vi "CalculateResidual.vi"(6 "calc cache":variant, 7 "Feature":T1, 8 "error in (no error)":errorcluster, 9 "Speed (RPM)":dbl, 10 "Channel":T3, 11 "Data":waveform(sgl)) -> (0 "error out":errorcluster, 3 "Residual [EU RMS]":dbl, 4 "calc cache out":variant)   [LabVIEW 2017, in "AnalysisHelper.lvlib"]
uses:
  <vilib>/addons/InsightCM/Utilities/Analysis/Shared/AnalysisHelper.lvlib
  <vilib>/addons/InsightCM/Utilities/Analysis/Shared/controls/Channel.ctl
  <vilib>/addons/InsightCM/Utilities/Analysis/Shared/controls/SpeedType.ctl
  <vilib>/addons/InsightCM/Utilities/Analysis/Shared/controls/Feature.ctl
  <vilib>/addons/InsightCM/Utilities/Analysis/Shared/controls/AmplitudeScale.ctl
  <vilib>/addons/InsightCM/Utilities/Analysis/Shared/controls/BandConfig.ctl
  <vilib>/addons/InsightCM/Utilities/Analysis/Shared/controls/BandDomain.ctl
  <vilib>/addons/InsightCM/Utilities/Analysis/Shared/controls/BandCalculation.ctl
  <vilib>/addons/InsightCM/Utilities/Analysis/Vibration/VibrationAnalysisFunctions.lvlib
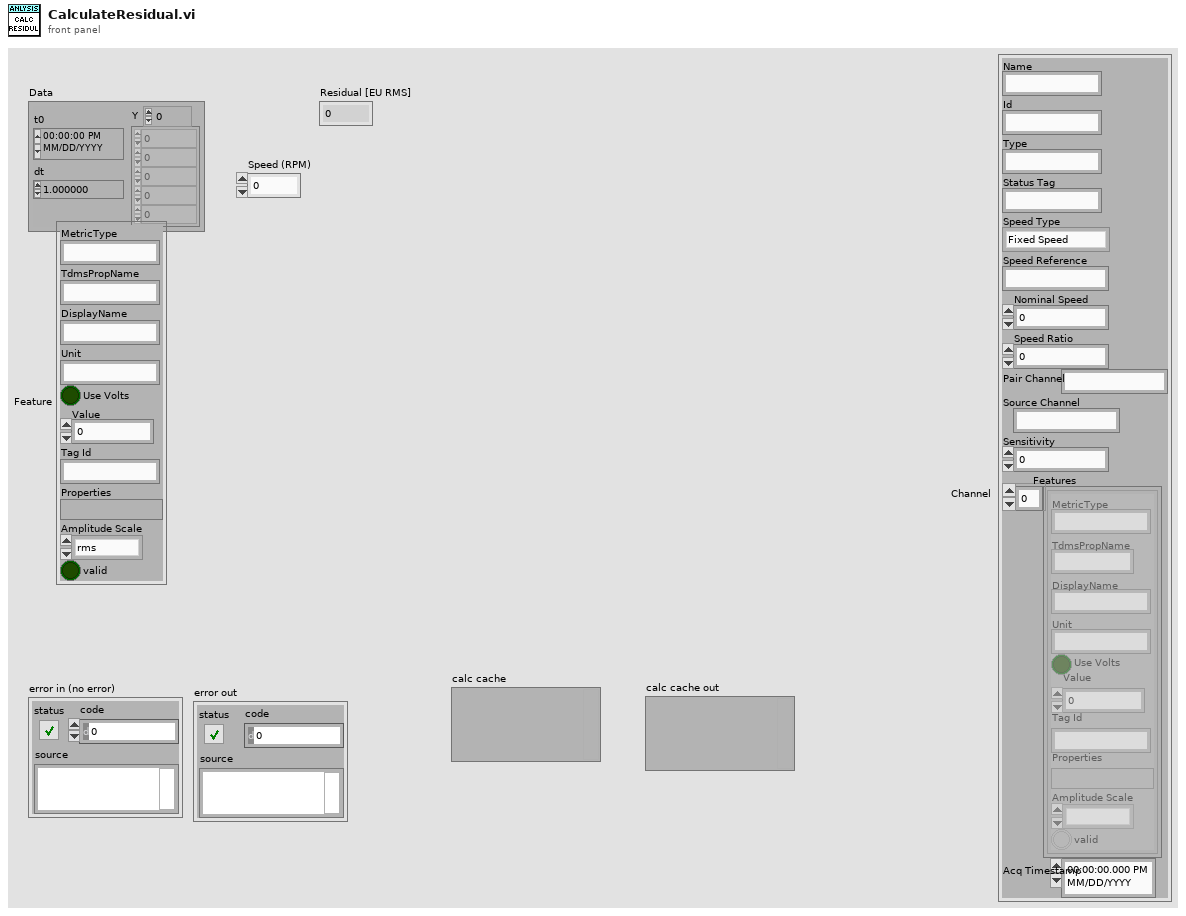
[diagram p1: front panel]
types:
  T1 = typedef "AnalysisHelper.lvlib/Feature.ctl" = cluster{"MetricType":string, "TdmsPropName":string, "DisplayName":string, "Unit":string, "Use Volts":bool, "Value":dbl, "Tag Id":string, "Properties":variant, "Amplitude Scale":T2, "valid":bool}
  T2 = typedef "AnalysisHelper.lvlib/AmplitudeScale.ctl" = enum16{"rms", "peak", "pk-pk"}
  T3 = typedef "AnalysisHelper.lvlib/Channel.ctl" = cluster{"Name":string, "Id":string, "Type":string, "Status Tag":string, "Speed Type":T4, "Speed Reference":string, "Nominal Speed":dbl, "Speed Ratio":dbl, "Pair Channel":string, "Source Channel":string, "Sensitivity":dbl, "Features":T1[], "Acq Timestamp":timestamp}
  T4 = typedef "AnalysisHelper.lvlib/SpeedType.ctl" = enum16{"Fixed Speed", "Tachometer"}
  T5 = typedef "AnalysisHelper.lvlib/BandConfig.ctl" = cluster{"High":dbl, "Low":dbl, "Domain":T6, "Calculation":T7}
  T6 = typedef "AnalysisHelper.lvlib/BandDomain.ctl" = enum16{"Frequency", "CPM", "Orders"}
  T7 = typedef "AnalysisHelper.lvlib/BandCalculation.ctl" = enum16{"Total", "Max", "Phase"}
  T8 = typedef "svc_Spectrum Info.ctl" = cluster{"channel name":string, "description":string, "x-axis units":T9, "spectral info":cluster{"spectrum type":T10, "linear/dB":enum16{"linear", "dB"}, "window":u16, "window size":i32, "FFT size":i32}, "engineering units":T11, "custom label":string, "dB reference [EU]":dbl, "peak units":enum16{"rms", "peak", "peak-peak"}, "weighting filter":T12, "spectral density?":bool, "unit label":string, "spectrum skewed?":bool, "complimentary spectrum units":T13}
  T9 = typedef "svc_X-Axis Units.ctl" = u16
  T10 = typedef "svc_Spectrum Type.ctl" = enum16{"FFT Spectrum [complex]", "Amplitude [Magnitude]", "Power [Magnitude^2]", "Cross Spectrum [complex]", "Frequency Response [Complex]"}
  T11 = typedef "svc_Engineering Units Text Ring.ctl" = u16
  T12 = typedef "svc_Weighting Filter Text Ring.ctl" = u16
  T13 = typedef "svc_Complimentary Spectrum Units.ctl" = enum16{"none", "radians", "degrees", "cycles", "imaginary"}
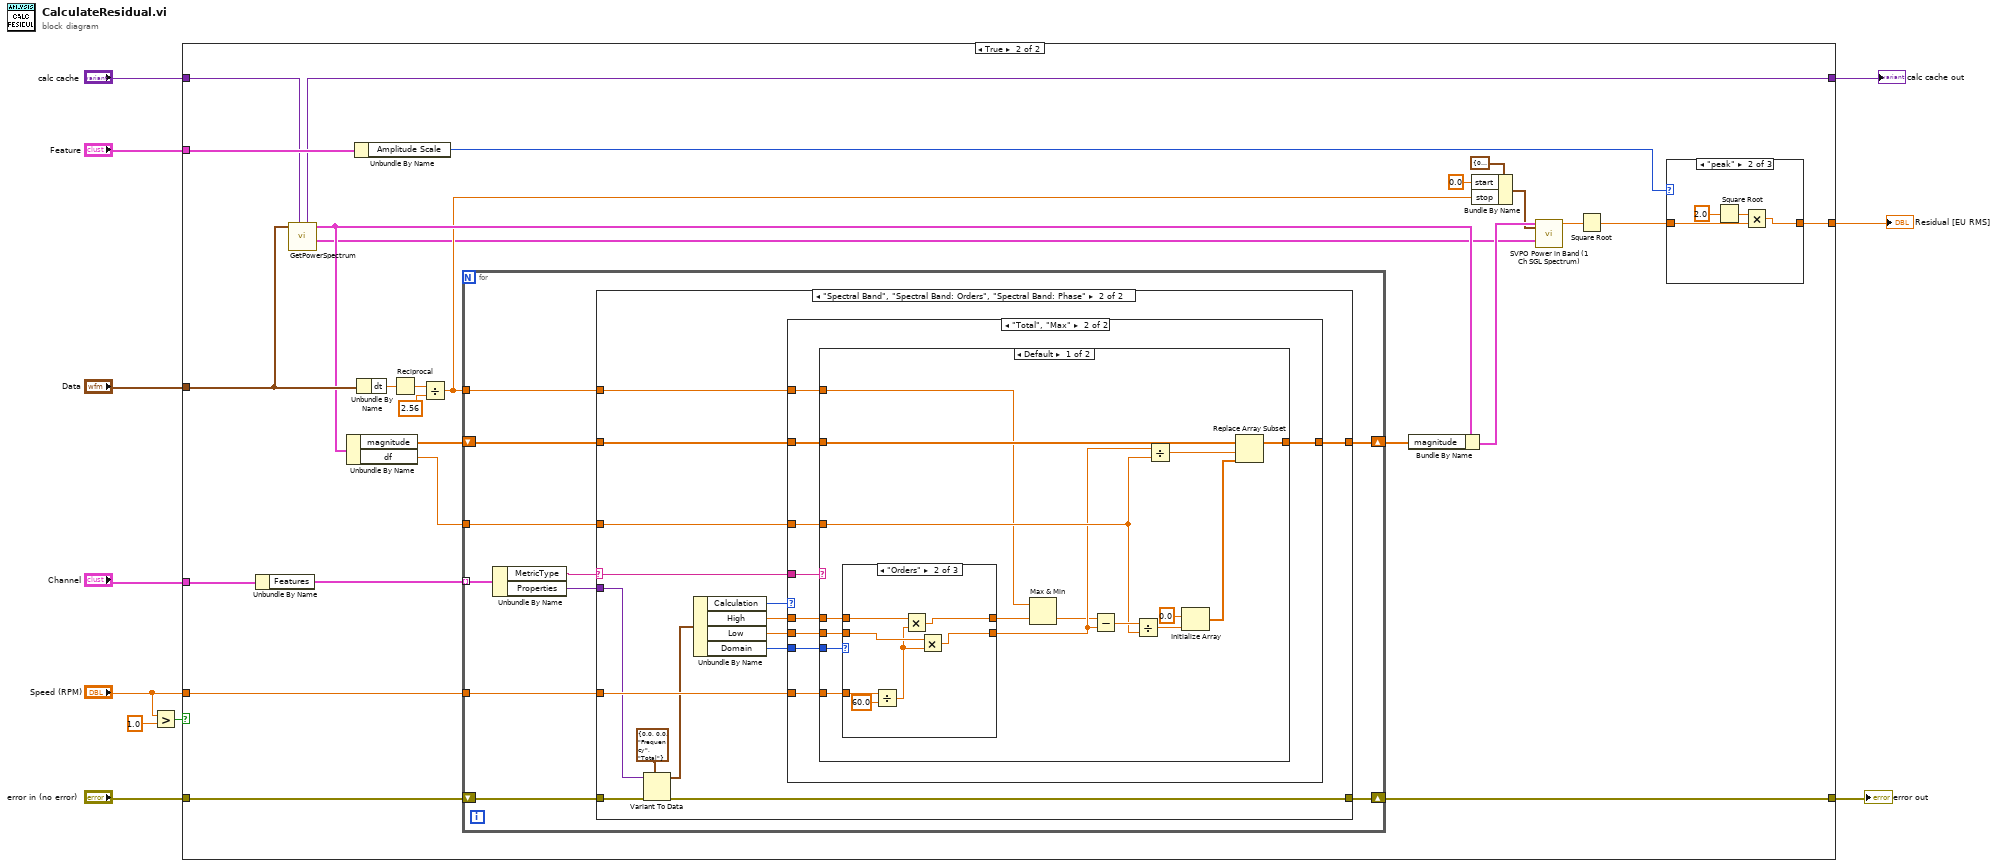
[diagram p0: block diagram]
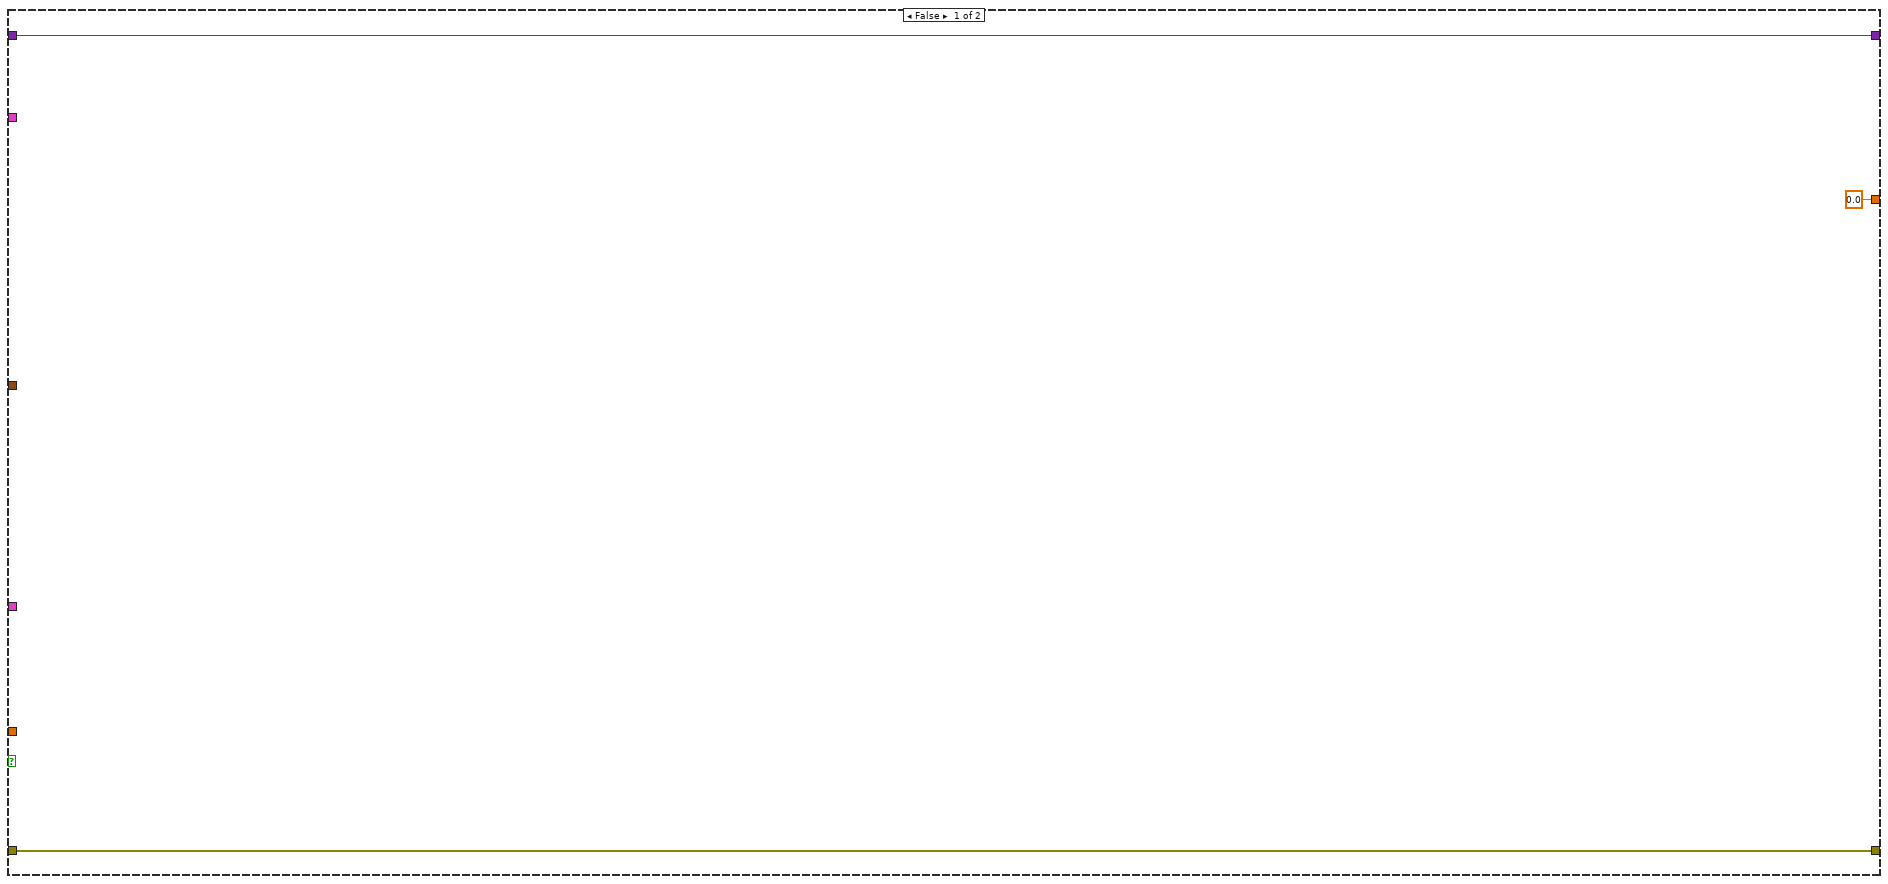
[diagram p2: hidden frame]
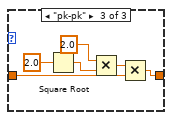
[diagram p4: hidden frame]
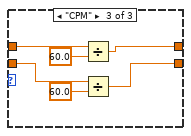
[diagram p8: hidden frame]
diagram:
  n1 = Greater?(x="Speed (RPM)", y=1.0) -> (0:w3:bool)
  n2 = case shown="True" w3 {
    tunnel: "Speed (RPM)" -> [_ w39]
    tunnel: "Data" -> [_ w38]
    tunnel: "error in (no error)" -> [w13 w28]
    tunnel: "Channel" -> [_ w27]
    tunnel: "Feature" -> [_ w25]
    tunnel: [sgl 0.0 w24] -> w7
    tunnel: "calc cache" -> [w12 w18]
    tunnel: [w13 w17] -> w5
    tunnel: [w12 w15] -> w1
    frame False {
    }
    frame True {
      n3 = Unbundle By Name(w27) -> ("Features"=w26:T1[])
      n4 = call <vilib>:"GetPowerSpectrum.vi"("calc cache"=w18, "Waveform"=w38) -> ("spectrum info"=w20:T8, "power spectrum [EU^2 rms]"=w34:cluster{"f0":dbl, "df":dbl, "magnitude":sgl[]}, "calc cache out"=w15:variant)  [unwired: 7 in]
      n5 = Unbundle By Name(w34) -> ("magnitude"=w32:sgl[], "df"=w40:dbl)
      n6 = Unbundle By Name(w25) -> ("Amplitude Scale"=w23:T2)
      n7 = Unbundle By Name(w38) -> ("dt"=w37:dbl)
      n8 = Reciprocal(x=w37) -> (1/x=w36:dbl)
      n9 = Divide(x=w36, y=2.56) -> (x/y=w29:dbl)
      n10 = for {
        tunnel: w26 -> [w61] mode=indexing
        shift-right: [w59] -> w33
        shift-left: w32 -> [w58]
        tunnel: w40 -> [w57]
        tunnel: w39 -> [w56]
        tunnel: w29 -> [w55]
        shift-right: [w53] -> w17
        shift-left: w28 -> [w54]
        n11 = Unbundle By Name(w61) -> ("MetricType"=w60:string, "Properties"=w52:variant)
        n12 = case shown="\"Spectral Band\", \"Spectral Band: Orders\", \"Spectral Band: Phase\"" w60 {
          selector: w60 -> [_ w70]
          tunnel: [w63 w78] -> w59
          tunnel: w58 -> [w63 w77]
          tunnel: w57 -> [_ w76]
          tunnel: w56 -> [_ w75]
          tunnel: w55 -> [_ w74]
          tunnel: w54 -> [w62 w66]
          tunnel: [w62 w65] -> w53
          tunnel: w52 -> [_ w64]
          frame "False", Default {
          }
          frame "Spectral Band", "Spectral Band: Orders", "Spectral Band: Phase" {
            n13 = Variant To Data(error in=w66, type=T5 {"High"=0.0, "Low"=0.0, "Domain"=enum."Frequency", "Calculation"=enum."Total"} ("SpectralBand"), Variant=w64) -> (data=w72:T5, error out=w65:errorcluster)
            n14 = Unbundle By Name(w72) -> ("Calculation"=w71:T7, "High"=w69:dbl, "Low"=w68:dbl, "Domain"=w67:T6)
            n15 = case shown="\"Total\", \"Max\"" w71 {
              tunnel: [w79 w88] -> w78
              tunnel: w77 -> [w79 w87]
              tunnel: w69 -> [_ w86]
              tunnel: w68 -> [_ w85]
              tunnel: w67 -> [_ w84]
              tunnel: w76 -> [_ w83]
              tunnel: w75 -> [_ w82]
              tunnel: w74 -> [_ w81]
              tunnel: w70 -> [_ w80]
              frame "Phase" {
              }
              frame "Total", "Max" {
                n16 = case shown="Default" w80 {
                  tunnel: [w89 w120] -> w88
                  tunnel: w87 -> [w104 w120]
                  tunnel: w86 -> [w100 _]
                  tunnel: w85 -> [w99 _]
                  tunnel: w84 -> [w101 _]
                  tunnel: w83 -> [w96 _]
                  tunnel: w82 -> [w93 _]
                  tunnel: w81 -> [w92 _]
                  frame Default {
                    n17 = case shown="\"Orders\"" w101 {
                      tunnel: w100 -> [w106 w113 w119]
                      tunnel: w99 -> [w105 w109 w115]
                      tunnel: [w106 w110 w116] -> w91
                      tunnel: [w105 w107 w114] -> w95
                      tunnel: w93 -> [_ w112 _]
                      frame "Frequency" {
                      }
                      frame "Orders" {
                        n18 = Divide(x=w112, y=60.0) -> (x/y=w108:dbl)
                        n19 = Multiply(x=w113, y=w108) -> (x*y=w110:dbl)
                        n20 = Multiply(x=w109, y=w108) -> (x*y=w107:dbl)
                      }
                      frame "CPM" {
                        n21 = Divide(x=w119, y=60.0) -> (x/y=w116:dbl)
                        n22 = Divide(x=w115, y=60.0) -> (x/y=w114:dbl)
                      }
                    }
                    n23 = Max & Min(x=w92, y=w91) -> (min(x,y)=w90:dbl)  [unwired: 1 out]
                    n24 = Subtract(x=w90, y=w95) -> (x-y=w98:dbl)
                    n25 = Divide(x=w98, y=w96) -> (x/y=w97:dbl)
                    n26 = Divide(x=w95, y=w96) -> (x/y=w94:dbl)
                    n27 = Initialize Array(sgl 0.0 ("element"), w97) -> (w102:sgl[])
                    n28 = Replace Array Subset(array=w104, new element=w102, index=w94) -> (w89:sgl[])
                  }
                  frame "SpectralBand: Residual" {
                  }
                }
              }
            }
          }
        }
      }
      n29 = Bundle By Name(cluster=w34, "magnitude"=w33) -> (w22:cluster{"f0":dbl, "df":dbl, "magnitude":sgl[]})
      n30 = Bundle By Name(cluster=cluster{"start":dbl, "stop":dbl} {"start"=0.0, "stop"=1000.0} ("range"), "start"=0.0, "stop"=w29) -> (w21:cluster{"start":dbl, "stop":dbl})
      n31 = call <vilib>:"SVPO Power in Band (1 Ch SGL Spectrum).vi"("spectrum [EU^2 rms]"=w22, "range"=w21, "spectrum info"=w20) -> ("power in band [EU^2 rms]"=w19:dbl)  [unwired: 16 in]
      n32 = Square Root(x=w19) -> (sqrt(x)=w16:dbl)
      n33 = case shown="\"peak\"" w23 {
        tunnel: w16 -> [w41 w45 w51]
        tunnel: [w41 w44 w50] -> w24
        frame "rms", Default {
        }
        frame "peak" {
          n34 = Square Root(x=sgl 2.0) -> (sqrt(x)=w43:sgl)
          n35 = Multiply(x=w43, y=w45) -> (x*y=w44:dbl)
        }
        frame "pk-pk" {
          n36 = Square Root(x=sgl 2.0) -> (sqrt(x)=w47:sgl)
          n37 = Multiply(x=sgl 2.0, y=w47) -> (x*y=w48:sgl)
          n38 = Multiply(x=w48, y=w51) -> (x*y=w50:dbl)
        }
      }
    }
  }
  "Residual [EU RMS]" <- w7
  "error out" <- w5
  "calc cache out" <- w1
